vi "Set Measurement Type.vi"(8 "error in (no error)":errorcluster, 10 "Measurement Type":T1=10 items=["Continuity", "Current AC", "Current DC", "Diode", "Frequency", "Resistance 4-wire", "Period", "Resistance 2-wire", "Temperature", "Voltage AC", "Voltage DC", "Voltage DC Ratio", "Capacitance"], 11 "34401 in":refnum<class "34401.lvclass">) -> (0 "error out":errorcluster, 3 "34401 out":refnum<class "34401.lvclass">)   [LabVIEW 2018, in "34401.lvlib" / "34401.lvclass"]
doc: "This Overrides is meant to be used/called from the 'Set Measurements Properties.vi' Method where other properties are given values."
uses:
  34401.lvclass
  PPLs/DMM/Parent/DMM.lvlibp/Custom Controls/Measurement Type.ctl
  34401.lvclass/34401.ctl
  <instrlib>/Agilent 34401/Agilent 34401.lvlib
  PPLs/DMM/Parent/DMM.lvlibp/DMM.lvclass
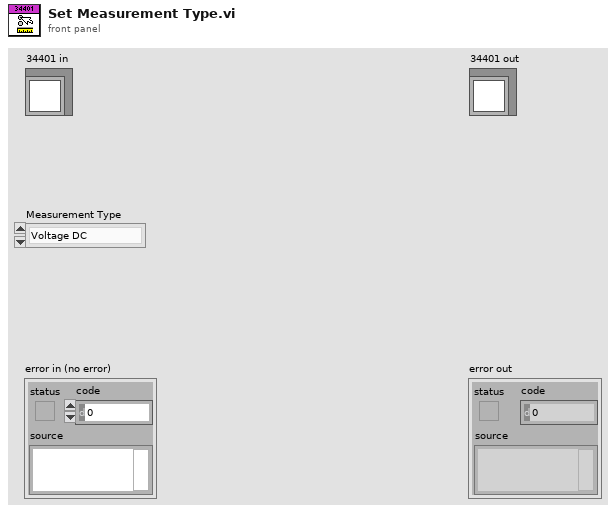
[diagram p1: front panel]
types:
  T1 = typedef "DMM.lvlibp/DMM.lvclass/Measurement Type.ctl" = u32
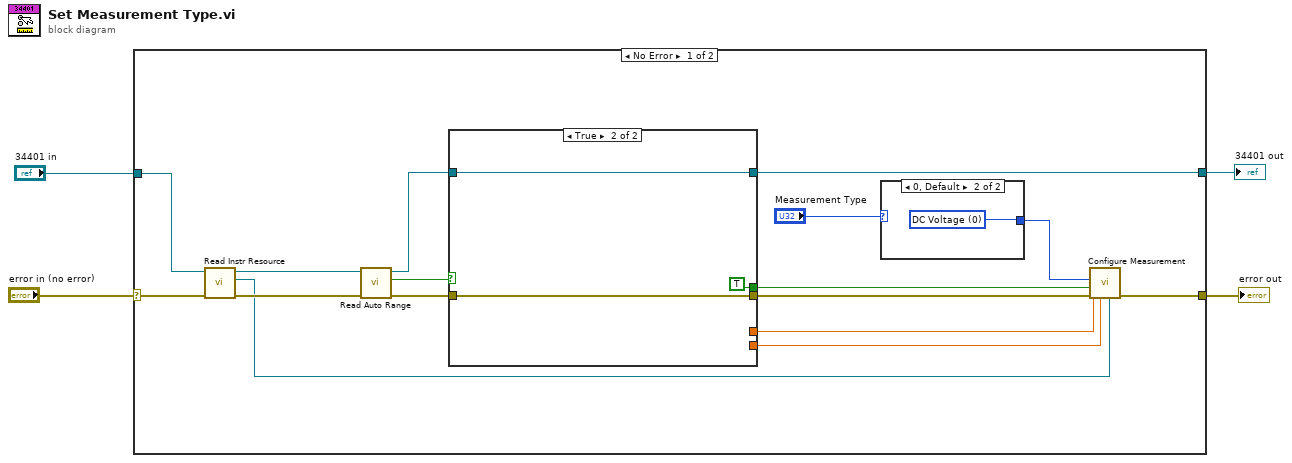
[diagram p0: block diagram]
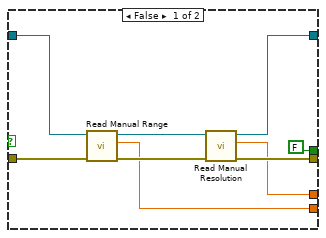
[diagram p2: hidden frame]
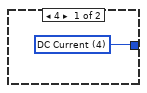
[diagram p3: hidden frame]
diagram:
  n1 = case shown="No Error" "error in (no error)" {
    selector: "error in (no error)" -> [w9 w35]
    tunnel: "34401 in" -> [w7 w36]
    tunnel: [w16 w36] -> w2
    tunnel: [w10 w35] -> w1
    frame No Error {
      n2 = call "Read Instr Resource.vi"("error in (no error)"=w9, "34401 in"=w7) -> ("error out"=w8:errorcluster, "Instr Resource"=w5:refnum<visa-resource-name>, "34401 out"=w6:refnum<class "34401.lvclass">)  [unwired: 7 in]
      n3 = call "Read Auto Range.vi"("error in (no error)"=w8, "34401 in"=w6) -> ("error out"=w15:errorcluster, "Auto Range"=w17:bool, "34401 out"=w18:refnum<class "34401.lvclass">)  [unwired: 7 in]
      n4 = case shown="True" w17 {
        tunnel: w18 -> [w25 w32]
        tunnel: [w23 w32] -> w16
        tunnel: w15 -> [w29 w31]
        tunnel: [FALSE TRUE] -> w14
        tunnel: [w27 w31] -> w13
        tunnel: [w26 _] -> w12
        tunnel: [w22 _] -> w11
        frame False {
          n5 = call "Read Manual Range.vi"("error in (no error)"=w29, "34401 in"=w25) -> ("error out"=w28:errorcluster, "Manual Range"=w26:dbl, "34401 out"=w24:refnum<class "34401.lvclass">)  [unwired: 7 in]
          n6 = call "Read Manual Resolution.vi"("error in (no error)"=w28, "34401 in"=w24) -> ("error out"=w27:errorcluster, "Manual Resolution"=w22:dbl, "34401 out"=w23:refnum<class "34401.lvclass">)  [unwired: 7 in]
        }
        frame True {
        }
      }
      n7 = case shown="0, Default" "Measurement Type" {
        tunnel: [w33 w34] -> w19
        frame 4 {
          w33 = u16 4 items=["DC Voltage", "AC Voltage", "2 - Wire Resistance", "4 - Wire Resistance", "DC Current", "AC Current", "Frequency", "Period", "Continuity", "Diode Checking", "VDC:VDC Ratio", "Temperature", "Capacitance"] ("Function (0: DC Voltage)")
        }
        frame 0, Default {
          w34 = u16 0 items=["DC Voltage", "AC Voltage", "2 - Wire Resistance", "4 - Wire Resistance", "DC Current", "AC Current", "Frequency", "Period", "Continuity", "Diode Checking", "VDC:VDC Ratio", "Temperature", "Capacitance"] ("Function (0: DC Voltage)")
        }
      }
      n8 = call <instrlib>:"Configure Measurement.vi"("Manual Range (1.00)"=w12, "Manual Resolution (5.5 Digits)"=w11, "error in (no error)"=w13, "Enable Auto Range (T: Enable)"=w14, "Function (0: DC Voltage)"=w19, "VISA resource name"=w5) -> ("error out"=w10:errorcluster)  [unwired: 4 in, 1 out]
    }
    frame Error {
    }
  }
  "error out" <- w1
  "34401 out" <- w2
